vi "merFISH_format_task_for_TDMS.vi"(4 "Task":T1, 5 "error in":errorcluster, 6 "setup state":i32[](array[numeric]), 7 "Task number":i32, 8 "tdms file":refnum<k34>) -> (0 "error out":errorcluster, 1 "setup state out":i32[](array[numeric]), 2 "Next task number":i32, 3 "tdms file out":refnum<k34>)   [LabVIEW 2015]
uses:
  CONTROLS/Q_main_element.ctl
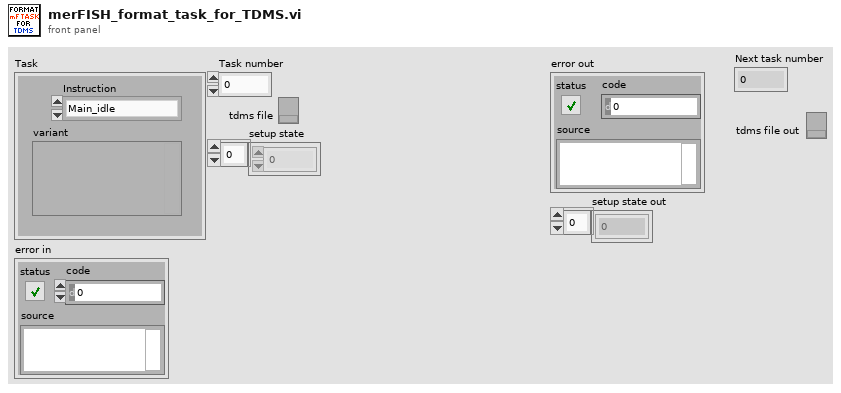
[diagram p1: front panel]
types:
  T1 = typedef "Q_main_element.ctl" = cluster{"variant":variant, "Instruction":enum16{"Main_idle", "Main_initialize", "Main_initialize_TDMS", "Main_initialize_Queue", "Main_error", "Main_DAQ_initialization_results", "Main_ASI_initialization_results", "Main_Piezo_initialization_results", "Main_Valve_initialization_results", "Main_Pump_initialization_results", "Main_CAMERA_initialization_results", "Main_FPGA_initialization_results", "Main_DAQ_error", "Main_ASI_error", "Main_Piezo_error", "Main_CAMERA_error", "Main_Valve_error", "Main_Pump_error", "Main_FPGA_error", "Main_start_acquiring", "Main_not_acquiring", "Main_acquiring", "Main_stop_acquiring", "Main_change_exposure", "Main_change_z_scan_parameters", "Main_define_ROI", "Main_define_mosaic", "Main_read_kinetic_time", "Main_cooler", "Main_read_temperature", "Main_save_XY", "Main_load_XY", "Main_discard_XY", "Main_move_to_XY", "Main_measure_QPD", "Main_autofocus_calibration", "Main_autofocus_initialization", "Main_autofocus_stop", "Main_save_PID", "Main_change_H_valve_position", "Main_two_way_valve", "Main_save_movie", "Main_init_single_scan", "Main_single_scan", "Main_stop_single_scan", "Main_merFISH_illumination_parameters", "Main_merFISH_buffer_probe_list", "Main_merFISH_injections_procedure", "Main_merFISH_save_setpoint", "Main_merFISH_DAPI_parameters", "Main_merFISH_Brightfield_parameters", "Main_merFISH_save_embryo_ROI", "Main_merFISH_init", "Main_merFISH_resume", "Main_merFISH_start_autofocus", "Main_merFISH_open_close_valve_merFISH", "Main_merFISH_open_close_valve_photobleaching", "Main_merFISH_hybridization", "Main_merFISH_move_to_ROI", "Main_merFISH_wait_stabilization", "Main_merFISH_move_to_REF", "Main_merFISH_scan", "Main_merFISH_photobleaching_injection", "Main_merFISH_photobleaching", "Main_merFISH_send_email", "Main_merFISH_close", "Main_STOP"}}
  T2 = enum16{"Main_idle", "Main_initialize", "Main_initialize_TDMS", "Main_initialize_Queue", "Main_error", "Main_DAQ_initialization_results", "Main_ASI_initialization_results", "Main_Piezo_initialization_results", "Main_Valve_initialization_results", "Main_Pump_initialization_results", "Main_CAMERA_initialization_results", "Main_FPGA_initialization_results", "Main_DAQ_error", "Main_ASI_error", "Main_Piezo_error", "Main_CAMERA_error", "Main_Valve_error", "Main_Pump_error", "Main_FPGA_error", "Main_start_acquiring", "Main_not_acquiring", "Main_acquiring", "Main_stop_acquiring", "Main_change_exposure", "Main_change_z_scan_parameters", "Main_define_ROI", "Main_define_mosaic", "Main_read_kinetic_time", "Main_cooler", "Main_read_temperature", "Main_save_XY", "Main_load_XY", "Main_discard_XY", "Main_move_to_XY", "Main_measure_QPD", "Main_autofocus_calibration", "Main_autofocus_initialization", "Main_autofocus_stop", "Main_save_PID", "Main_change_H_valve_position", "Main_two_way_valve", "Main_save_movie", "Main_init_single_scan", "Main_single_scan", "Main_stop_single_scan", "Main_merFISH_illumination_parameters", "Main_merFISH_buffer_probe_list", "Main_merFISH_injections_procedure", "Main_merFISH_save_setpoint", "Main_merFISH_DAPI_parameters", "Main_merFISH_Brightfield_parameters", "Main_merFISH_save_embryo_ROI", "Main_merFISH_init", "Main_merFISH_resume", "Main_merFISH_start_autofocus", "Main_merFISH_open_close_valve_merFISH", "Main_merFISH_open_close_valve_photobleaching", "Main_merFISH_hybridization", "Main_merFISH_move_to_ROI", "Main_merFISH_wait_stabilization", "Main_merFISH_move_to_REF", "Main_merFISH_scan", "Main_merFISH_photobleaching_injection", "Main_merFISH_photobleaching", "Main_merFISH_send_email", "Main_merFISH_close", "Main_STOP"}
  T3 = cluster{"ROI #":i32, "Probe #":i32, "Folder# ":i32, "Embryo #":i32}
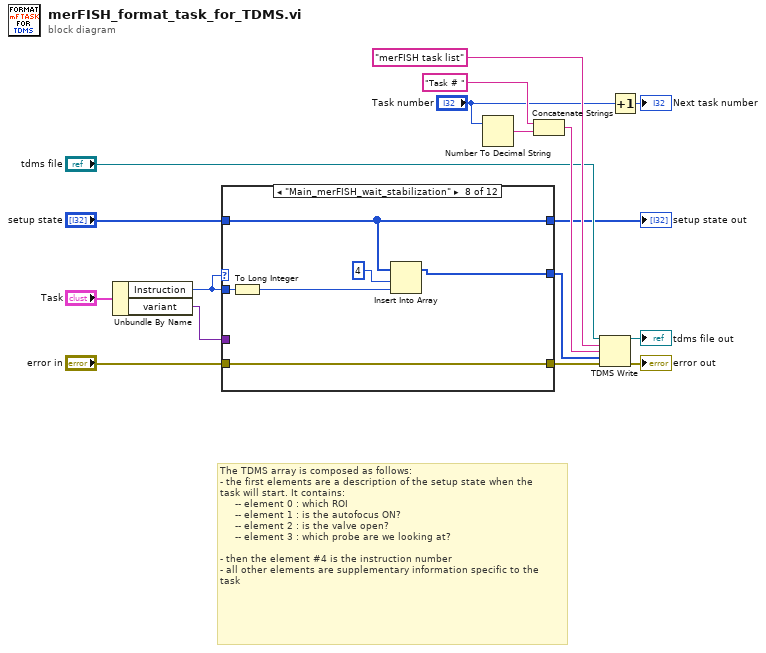
[diagram p0: block diagram]
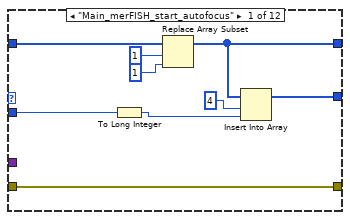
[diagram p2: hidden frame]
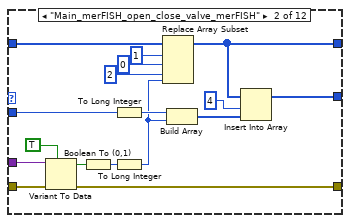
[diagram p3: hidden frame]
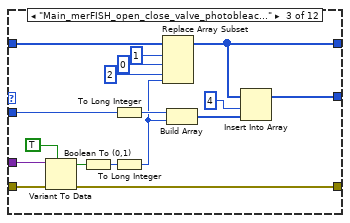
[diagram p4: hidden frame]
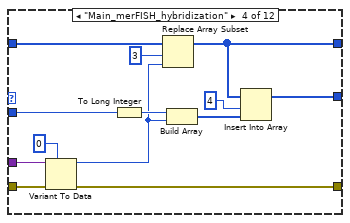
[diagram p5: hidden frame]
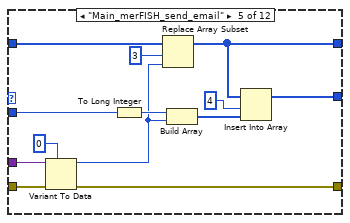
[diagram p6: hidden frame]
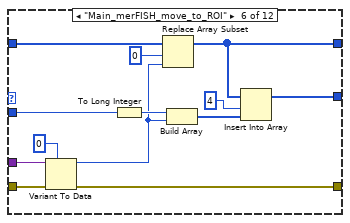
[diagram p7: hidden frame]
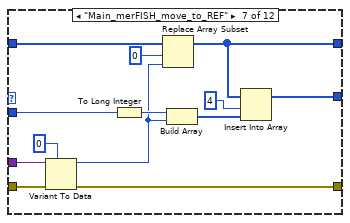
[diagram p8: hidden frame]
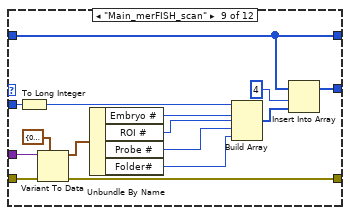
[diagram p9: hidden frame]
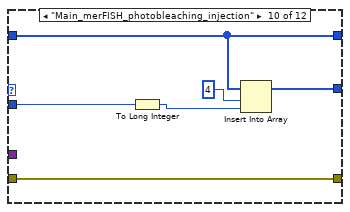
[diagram p10: hidden frame]
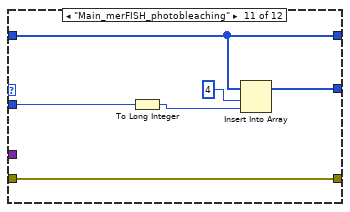
[diagram p11: hidden frame]
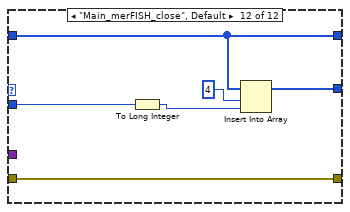
[diagram p12: hidden frame]
diagram:
  # "The TDMS array is composed as follows:\n- the first elements are a description of the setup state when the \ntask will start. It contains:\n     -- element 0 : which ROI\n     -- element 1 : is the autofocus ON?\n     -- element 2 : is the valve open?\n     -- element 3 : which probe are we looking at?\n\n- then the element #4 is the instruction number\n- all other elements are supplementary information specific to the\ntask"
  n1 = Unbundle By Name("Task") -> ("Instruction"=w12:T2, "variant"=w11:variant)
  n2 = case shown="\"Main_merFISH_wait_stabilization\"" w12 {
    tunnel: w12 -> [w26 w43 w60 w73 w86 w99 w112 w116 w129 w137 w143 w149]
    tunnel: [w22 w31 w48 w64 w77 w90 w103 w117 w132 w138 w144 w150] -> w8
    tunnel: w11 -> [_ w41 w58 w71 w84 w97 w110 _ w128 _ _ _]
    tunnel: "error in" -> [w19 w39 w56 w70 w83 w96 w109 w114 w127 w135 w141 w147]
    tunnel: [w19 w36 w53 w69 w82 w95 w108 w114 w126 w135 w141 w147] -> w9
    tunnel: "setup state" -> [w25 w35 w52 w68 w81 w94 w107 w115 w124 w136 w142 w148]
    tunnel: [w21 w30 w47 w61 w74 w87 w100 w115 w124 w136 w142 w148] -> w1
    frame "Main_merFISH_start_autofocus" {
      n3 = To Long Integer(number=w26) -> (32bit integer=w20:i32)
      n4 = Replace Array Subset(array=w25, new element=1 ("new element/subarray"), index=1) -> (w21:i32[])
      n5 = Insert Into Array(array=w21, index=4, new element=w20) -> (w22:i32[])
    }
    frame "Main_merFISH_open_close_valve_merFISH" {
      n6 = Variant To Data(error in=w39, type=TRUE, Variant=w41) -> (data=w38:bool, error out=w36:errorcluster)
      n7 = Boolean To (0,1)(Boolean=w38) -> (0, 1=w37:i16)
      n8 = To Long Integer(number=w43) -> (32bit integer=w42:i32)
      n9 = To Long Integer(number=w37) -> (32bit integer=w29:i32)
      n10 = Replace Array Subset(array=w35, new element #1=0 ("new element/subarray"), index #1=1 ("index"), new element #2=w29, index #2=2 ("index")) -> (w30:i32[])
      n11 = Build Array(w42, w29) -> (w33:i32[])
      n12 = Insert Into Array(array=w30, index=4, new element=w33) -> (w31:i32[])
    }
    frame "Main_merFISH_open_close_valve_photobleaching" {
      n13 = Variant To Data(error in=w56, type=TRUE, Variant=w58) -> (data=w55:bool, error out=w53:errorcluster)
      n14 = Boolean To (0,1)(Boolean=w55) -> (0, 1=w54:i16)
      n15 = To Long Integer(number=w60) -> (32bit integer=w59:i32)
      n16 = To Long Integer(number=w54) -> (32bit integer=w46:i32)
      n17 = Replace Array Subset(array=w52, new element #1=0 ("new element/subarray"), index #1=1 ("index"), new element #2=w46, index #2=2 ("index")) -> (w47:i32[])
      n18 = Build Array(w59, w46) -> (w50:i32[])
      n19 = Insert Into Array(array=w47, index=4, new element=w50) -> (w48:i32[])
    }
    frame "Main_merFISH_hybridization" {
      n20 = Variant To Data(error in=w70, type=0, Variant=w71) -> (data=w62:i32, error out=w69:errorcluster)
      n21 = To Long Integer(number=w73) -> (32bit integer=w72:i32)
      n22 = Replace Array Subset(array=w68, new element=w62, index=3) -> (w61:i32[])
      n23 = Build Array(w72, w62) -> (w66:i32[])
      n24 = Insert Into Array(array=w61, index=4, new element=w66) -> (w64:i32[])
    }
    frame "Main_merFISH_send_email" {
      n25 = Variant To Data(error in=w83, type=0, Variant=w84) -> (data=w75:i32, error out=w82:errorcluster)
      n26 = To Long Integer(number=w86) -> (32bit integer=w85:i32)
      n27 = Replace Array Subset(array=w81, new element=w75, index=3) -> (w74:i32[])
      n28 = Build Array(w85, w75) -> (w79:i32[])
      n29 = Insert Into Array(array=w74, index=4, new element=w79) -> (w77:i32[])
    }
    frame "Main_merFISH_move_to_ROI" {
      n30 = Variant To Data(error in=w96, type=0, Variant=w97) -> (data=w88:i32, error out=w95:errorcluster)
      n31 = To Long Integer(number=w99) -> (32bit integer=w98:i32)
      n32 = Replace Array Subset(array=w94, new element=w88, index=0) -> (w87:i32[])
      n33 = Build Array(w98, w88) -> (w92:i32[])
      n34 = Insert Into Array(array=w87, index=4, new element=w92) -> (w90:i32[])
    }
    frame "Main_merFISH_move_to_REF" {
      n35 = Variant To Data(error in=w109, type=0, Variant=w110) -> (data=w101:i32, error out=w108:errorcluster)
      n36 = To Long Integer(number=w112) -> (32bit integer=w111:i32)
      n37 = Replace Array Subset(array=w107, new element=w101, index=0) -> (w100:i32[])
      n38 = Build Array(w111, w101) -> (w105:i32[])
      n39 = Insert Into Array(array=w100, index=4, new element=w105) -> (w103:i32[])
    }
    frame "Main_merFISH_wait_stabilization" {
      n40 = To Long Integer(number=w116) -> (32bit integer=w113:i32)
      n41 = Insert Into Array(array=w115, index=4, new element=w113) -> (w117:i32[])
    }
    frame "Main_merFISH_scan" {
      n42 = To Long Integer(number=w129) -> (32bit integer=w131:i32)
      n43 = Variant To Data(error in=w127, type=T3 {"ROI #"=0, "Probe #"=0, "Folder# "=0, "Embryo #"=0}, Variant=w128) -> (data=w130:T3, error out=w126:errorcluster)
      n44 = Unbundle By Name(w130) -> ("Embryo #"=w122:i32, "ROI #"=w121:i32, "Probe #"=w120:i32, "Folder#"=w119:i32)
      n45 = Build Array(w131, w122, w121, w120, w119) -> (w125:i32[])
      n46 = Insert Into Array(array=w124, index=4, new element=w125) -> (w132:i32[])
    }
    frame "Main_merFISH_photobleaching_injection" {
      n47 = To Long Integer(number=w137) -> (32bit integer=w134:i32)
      n48 = Insert Into Array(array=w136, index=4, new element=w134) -> (w138:i32[])
    }
    frame "Main_merFISH_photobleaching" {
      n49 = To Long Integer(number=w143) -> (32bit integer=w140:i32)
      n50 = Insert Into Array(array=w142, index=4, new element=w140) -> (w144:i32[])
    }
    frame "Main_merFISH_close", Default {
      n51 = To Long Integer(number=w149) -> (32bit integer=w146:i32)
      n52 = Insert Into Array(array=w148, index=4, new element=w146) -> (w150:i32[])
    }
  }
  "setup state out" <- w1
  n53 = Number To Decimal String(number="Task number") -> (decimal integer string=w17:string)  [unwired: 1 in]
  n54 = Concatenate Strings("Task # " ("string"), w17) -> (w15:string)
  n55 = TDMS Write(0:"tdms file", 5:"merFISH task list" ("group name in (Untitled)"), 7:w15, 9:w8, 11:w9) -> (4:→"tdms file out":refnum<k34>, 15:→"error out":errorcluster)  [unwired: 1 in, 2 out]
  n56 = Increment(x="Task number") -> (x+1=→"Next task number":i32)
